vi "Task Type.vi"(11 "AbortManager in":refnum<class "AbortManager.lvclass">) -> (2 "Task Type":string)   [LabVIEW 2020, in "Volatus.lvlib" / "AbortManager.lvclass"]
uses:
  AbortManager.lvclass
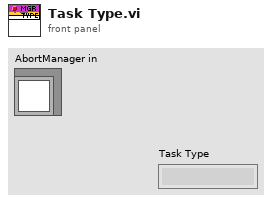
[diagram p1: front panel]
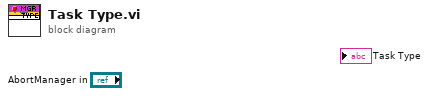
[diagram p0: block diagram]
diagram:
